vi "AppendChannels.vi"(1 "Append Channels":tag, 2 "Output Channels (input)":tag) -> (0 "Output Channels (output)":tag)   [LabVIEW 2009]
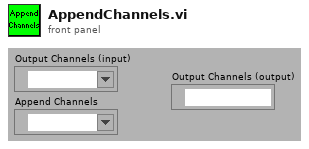
[diagram p1: front panel]
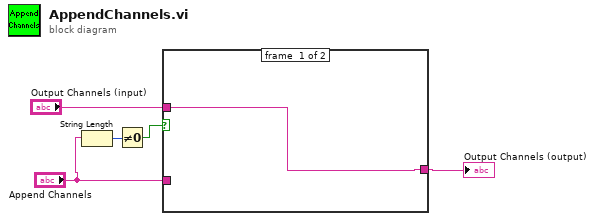
[diagram p0: block diagram]
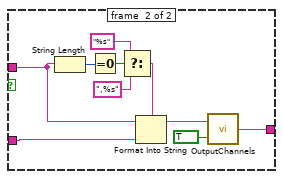
[diagram p2: hidden frame]
diagram:
  n1 = String Length(string="Append Channels") -> (length=w3:i32)
  n2 = Not Equal To 0?(x=w3) -> (x != 0?=w1:bool)
  n3 = case shown="True" w1 {
    tunnel: "Append Channels" -> [_ w11]
    tunnel: "Output Channels (input)" -> [w6 w8]
    tunnel: [w6 w7] -> w4
    frame #0 {
    }
    frame #1 {
      n4 = String Length(string=w8) -> (length=w12:i32)
      n5 = Equal To 0?(x=w12) -> (x = 0?=w16:bool)
      n6 = Select(t="%s" ("format string"), s=w16, f=",%s" ("format string")) -> (s? t:f=w13:string)
      n7 = Format Into String(format string=w13, initial string=w8, w11) -> (resulting string=w9:string)  [unwired: 1 in, 1 out]
      n8 = call "OutputChannels.vi"("Get/Set"=TRUE, "Output Channels (input)"=w9) -> ("Output Channels (output)"=w7:tag)
    }
  }
  "Output Channels (output)" <- w4
